vi "FTW-TransferClient-Initialize.vi"(0 "Transfer Client":refnum<class "FTW-TransferClient.lvclass">, 5 "Headers":T1[](array[typedef]), 11 "error in":errorcluster) -> (4 "Transfer Client out":refnum<class "FTW-TransferClient.lvclass">, 15 "error out":errorcluster)   [LabVIEW 2013, in "FTW-TransferClient.lvclass"]
uses:
  FTW-TransferClient.lvclass
  Collection/FTW-Collection-KeyValuePair.ctl
  FTW-TransferClient.lvclass/FTW-TransferClient.ctl
panel:
  # "Inputs"
  # "Outputs"
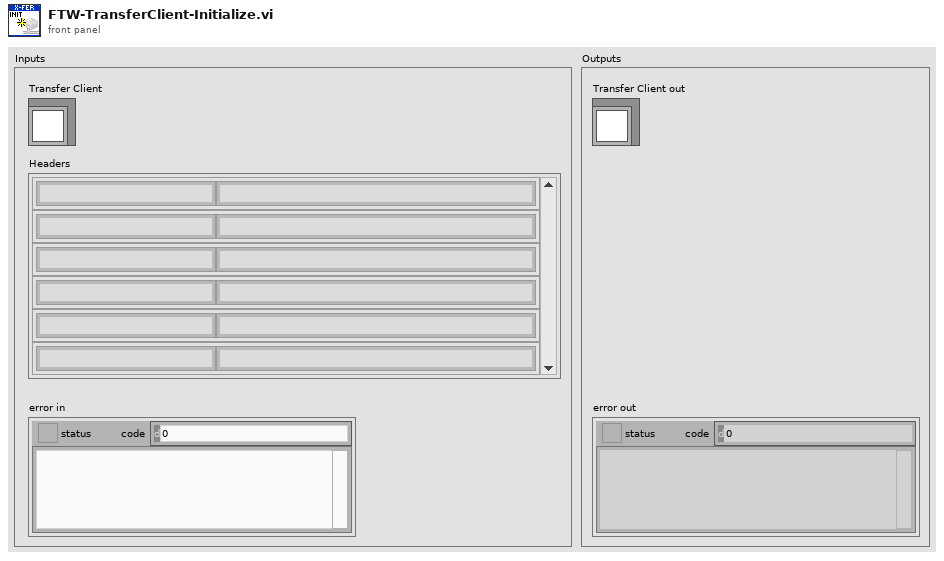
[diagram p1: front panel]
types:
  T1 = typedef "FTW-Collection-KeyValuePair.ctl" = cluster{"Key":string, "Value":string}
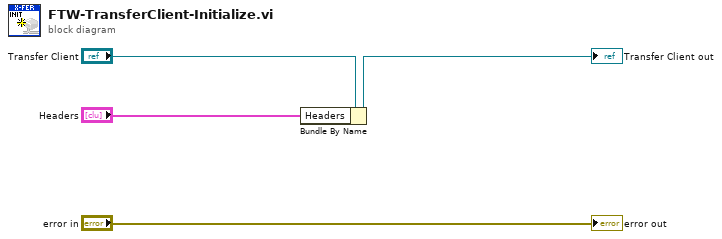
[diagram p0: block diagram]
diagram:
  n1 = Bundle By Name(cluster="Transfer Client", "Headers"="Headers") -> (→"Transfer Client out":refnum<class "FTW-TransferClient.lvclass">)
  "error out" <- "error in"
